vi "U3 Efunction Loop Example.vi"() -> (0 "error out":errorcluster)   [LabVIEW 2018]
panel:
  in  "stop":bool
  in  "Interval (ms)":u32=500
  out "FIO5 State In":bool
  in  "DAC0 Voltage":dbl format="%.3f"
  in  "FIO4 State Out":bool
  in  "FirstFound":bool=TRUE
  in  "Address":string="1"
  out "Error Message":string
  out "AIN0 Voltage":dbl format="%.6f"
  # "Sets DAC0, sets FIO4, reads AIN0, and reads FIO5."
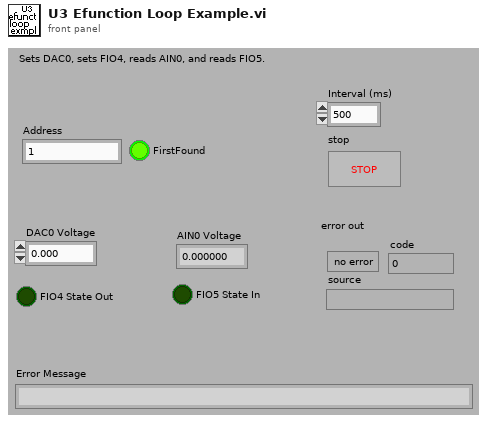
[diagram p1: front panel]
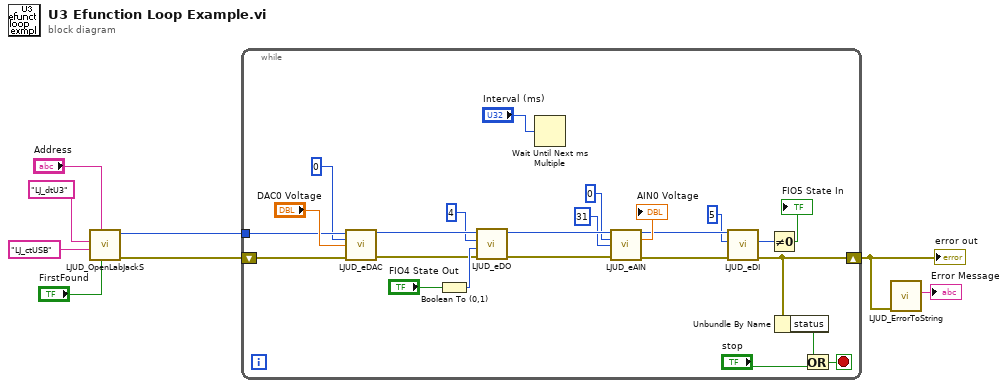
[diagram p0: block diagram]
diagram:
  n1 = call "LJUD_OpenLabJackS.vi"("FirstFound"="FirstFound", "Address"="Address", "ConnectionType"="LJ_ctUSB", "DeviceType"="LJ_dtU3") -> ("error out"=w1:errorcluster, "Handle"=w3:i32)  [unwired: 5 in, 1 out]
  n2 = while {
    shift-left: w1 -> [w10]
    shift-right: [w11] -> w2
    tunnel: w3 -> [w26]
    stop <- w13 stop-if-true
    n3 = call "LJUD_eDAC.vi"("Handle In"=w26, "Channel"=0, "Voltage"="DAC0 Voltage", "error in"=w10) -> ("Handle Out"=w24:i32, "error out"=w25:errorcluster)  [unwired: 10 in]
    n4 = Boolean To (0,1)(Boolean="FIO4 State Out") -> (0, 1=w30:i16)
    n5 = call "LJUD_eDO.vi"("error in"=w25, "State"=w30, "Channel"=4, "Handle In"=w24) -> ("error out"=w23:errorcluster, "Handle Out"=w22:i32)  [unwired: 6 in]
    n6 = Wait Until Next ms Multiple(millisecond multiple="Interval (ms)") -> ()  [unwired: 1 out]
    n7 = call "LJUD_eAIN.vi"("Handle In"=w22, "ChannelP"=0, "ChannelN"=31, "error in"=w23) -> ("Handle Out"=w17:i32, "Voltage"=→"AIN0 Voltage":dbl, "error out"=w27:errorcluster)  [unwired: 9 in]
    n8 = call "LJUD_eDI.vi"("error in"=w27, "Channel"=5, "Handle In"=w17) -> ("error out"=w11:errorcluster, "State"=w31:i32)  [unwired: 6 in, 1 out]
    n9 = Not Equal To 0?(x=w31) -> (x != 0?=→"FIO5 State In":bool)
    n10 = Unbundle By Name(w11) -> ("status"=w12:bool)
    n11 = Or(x=w12, y="stop") -> (x .or. y?=w13:bool)
  }
  "error out" <- w2
  n12 = call "LJUD_ErrorToString.vi"("error in"=w2) -> ("String"=→"Error Message":string)  [unwired: 10 in]
